vi "linlog.vi"(6 "CzyLog":dbl, 8 "Iteracja":dbl, 9 "pkt":dbl, 10 "max":dbl, 11 "min":dbl) -> (3 "częstotliwość":dbl)   [LabVIEW 2018]
doc: "Rozkłada punkty pomiarowe logarytmicznie lub liniowo."
uses:
  <vilib>/Analysis/1siggen.llb/Ramp Pattern by Samples.vi
  <vilib>/Analysis/NI_AALBase.lvlib
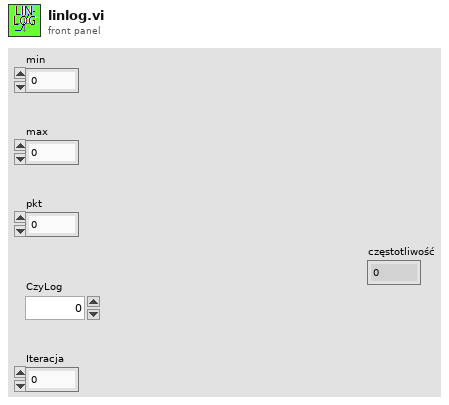
[diagram p1: front panel]
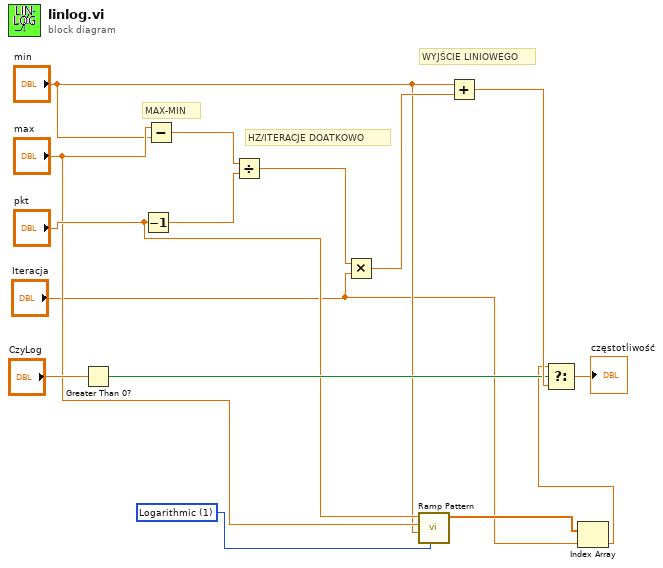
[diagram p0: block diagram]
diagram:
  w7 = u16 1 items=["Linear", "Logarithmic"] ("type")
  # "WYJŚCIE LINIOWEGO"
  # "HZ/ITERACJE DOATKOWO"
  # "MAX-MIN"
  n1 = Greater Than 0?(x="CzyLog") -> (x > 0?=w8:bool)
  n2 = Decrement(x="pkt") -> (x-1=w14:dbl)
  n3 = Subtract(x="max", y="min") -> (x-y=w15:dbl)
  n4 = Divide(x=w15, y=w14) -> (x/y=w13:dbl)
  n5 = Multiply(x=w13, y="Iteracja") -> (x*y=w12:dbl)
  n6 = call-poly <vilib>:"Ramp Pattern.vi"("type"=w7, "start"="min", "end"="max", "samples"="pkt") -> ("Ramp Pattern"=w3:dbl[])  [unwired: 6 in, 1 out]
  n7 = Add(x="min", y=w12) -> (x+y=w11:dbl)
  n8 = Index Array(array=w3, index="Iteracja") -> (element=w1:dbl)
  n9 = Select(t=w1, s=w8, f=w11) -> (s? t:f=→"częstotliwość":dbl)
